vi "SetWinSize.vi"(8 "error in (no error)":errorcluster, 9 "Width":u32, 10 "Height":u32, 11 "FolloWin in":refnum<class "FolloWin.lvclass">) -> (0 "error out":errorcluster, 3 "FolloWin out":refnum<class "FolloWin.lvclass">)   [LabVIEW 2023, in "FolloWin.lvclass"]
doc: "Resizes the FolloWin window."
uses:
  FolloWin.lvclass
  FolloWin.lvclass/FolloWin.ctl
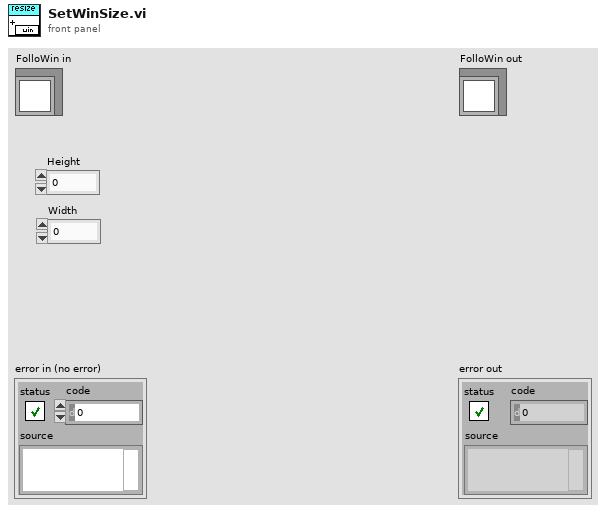
[diagram p1: front panel]
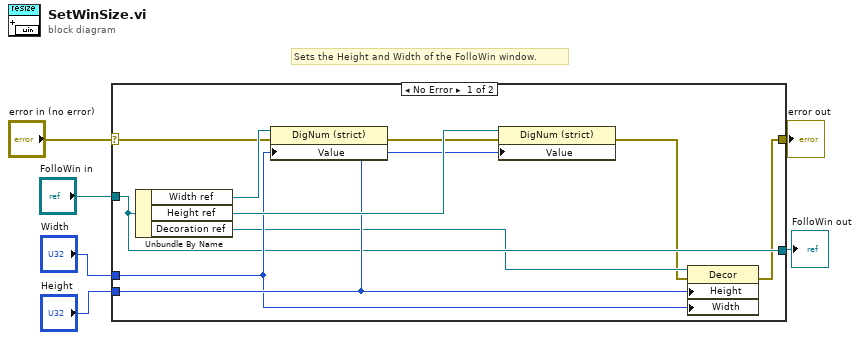
[diagram p0: block diagram]
diagram:
  # "Sets the Height and Width of the FolloWin window."
  n1 = case shown="No Error" "error in (no error)" {
    selector: "error in (no error)" -> [w14 w18]
    tunnel: [w9 w18] -> w5
    tunnel: [w10 w17] -> w3
    tunnel: "FolloWin in" -> [w10 w17]
    tunnel: "Height" -> [w12 _]
    tunnel: "Width" -> [w11 _]
    frame No Error {
      n2 = Unbundle By Name(w10) -> ("Width ref"=w16:refnum<vi>, "Height ref"=w15:refnum<vi>, "Decoration ref"=w8:refnum<vi>)
      n3 = property on="Property Node" class="DigNum (strict)"(reference=w16, error in=w14, "Value"=w11) -> (error out=w13:errorcluster)  [unwired: 1 out]
      n4 = property on="Property Node" class="DigNum (strict)"(reference=w15, error in=w13, "Value"=w12) -> (error out=w7:errorcluster)  [unwired: 1 out]
      n5 = property on="Property Node" class="Decor"(reference=w8, error in=w7, "Height"=w12, "Width"=w11) -> (error out=w9:errorcluster)  [unwired: 1 out]
    }
    frame Error {
    }
  }
  "error out" <- w5
  "FolloWin out" <- w3
